vi "Load_Position.vi"(4 "Relative?":bool, 6 "Error In":errorcluster, 7 "Position":i64, 8 "Node":u8=1, 9 "Serial In":refnum<visa-resource-name>) -> (0 "Error Out":errorcluster={"status"=TRUE, "code"=5000, "source"="Validate Command.vi<ERR>\nMotor Controller Error.\n\n\n<b>Complete call chain:</b>\n     Validate Command.vi\n     Load_Position.vi"}, 3 "Serial Out":refnum<visa-resource-name>)   [LabVIEW 2019, in "Faulhaber RS232.lvlib"]
uses:
  <instrlib>/Faulhaber RS232/Faulhaber RS232.lvlib
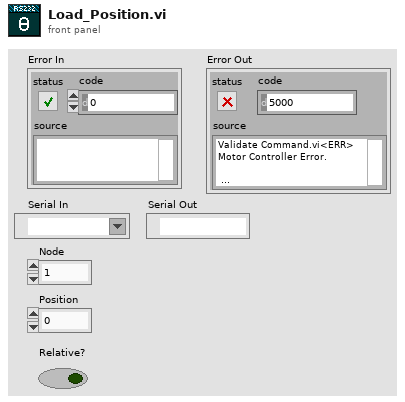
[diagram p1: front panel]
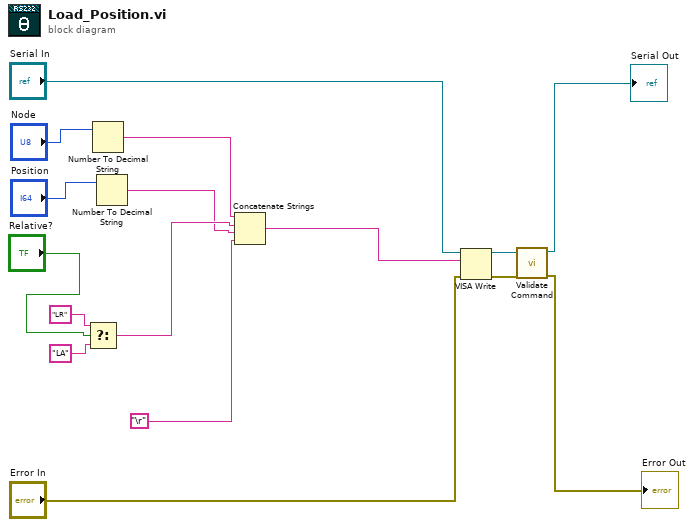
[diagram p0: block diagram]
diagram:
  n1 = Select(t="LR", s="Relative?", f="LA") -> (s? t:f=w9:string)
  n2 = Number To Decimal String(number="Node") -> (decimal integer string=w10:string)  [unwired: 1 in]
  n3 = Number To Decimal String(number="Position") -> (decimal integer string=w8:string)  [unwired: 1 in]
  n4 = Concatenate Strings(w10, w9, w8, "\r") -> (w7:string)
  n5 = VISA Write(VISA resource name="Serial In", write buffer=w7, error in (no error)="Error In") -> (VISA resource name out=w5:refnum<visa-resource-name>, error out=w4:errorcluster)  [unwired: 1 out]
  n6 = call <instrlib>:"Validate Command.vi"("error in (no error)"=w4, "Serial in"=w5) -> ("error out"=→"Error Out":errorcluster, "Serial Out"=→"Serial Out":refnum<visa-resource-name>)  [unwired: 3 in, 1 out]
